vi "欧姆龙PLC初始化FansTCP.vi"() -> (1 "data out":string, 2 "布尔":bool, 3 "TCP网络连接输出":refnum<k5>, 4 "打开TCP连接成功":bool)   [LabVIEW 2014]
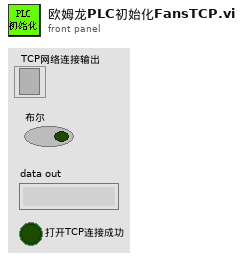
[diagram p1: front panel]
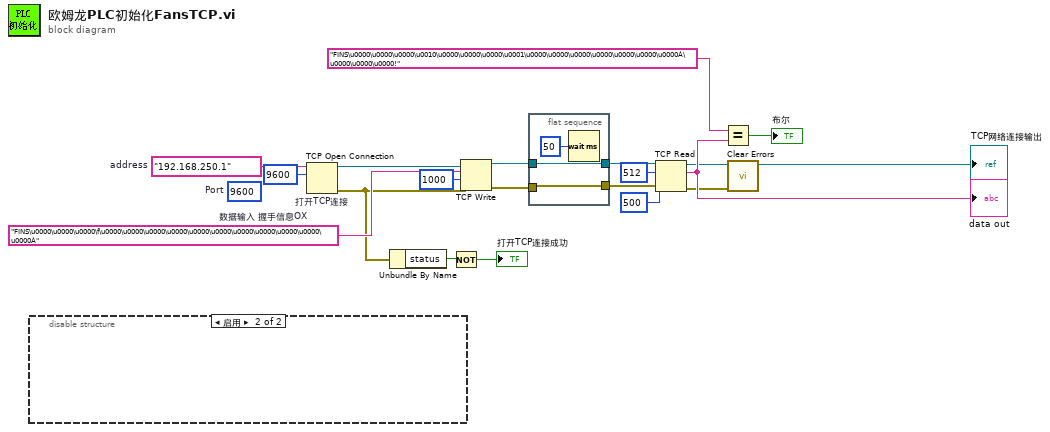
[diagram p0: block diagram]
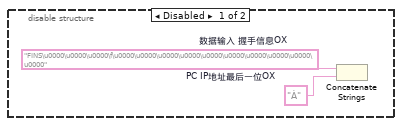
[diagram p2: hidden frame]
diagram:
  w15 = "FINS\u0000\u0000\u0000\f\u0000\u0000\u0000\u0000\u0000\u0000\u0000\u0000\u0000\u0000\u0000À"  # 数据输入 握手信息OX
  (unwired) 9600  # Port
  w2 = "192.168.250.1"  # address
  n1 = disable-structure shown="启用" {
    frame Disabled {
      w21 = "À"  # PC IP地址最后一位OX
      w20 = "FINS\u0000\u0000\u0000\f\u0000\u0000\u0000\u0000\u0000\u0000\u0000\u0000\u0000\u0000"  # 数据输入 握手信息OX
      n2 = Concatenate Strings(w20, w21) -> ()  [unwired: 1 out]
    }
    frame Enabled {
    }
  }
  n3 = TCP Open Connection "打开TCP连接"(address=w2, remote port or service name=u16 9600 ("远程端口或服务名称")) -> (connection ID=w6:refnum<k5>, error out=w7:errorcluster)  [unwired: 3 in]
  n4 = Unbundle By Name(w7) -> ("status"=w5:bool)
  n5 = Not(x=w5) -> (.not. x?=→"打开TCP连接成功":bool)
  n6 = TCP Write(connection ID=w6, data in=w15, error in (no error)=w7, 9:1000 ("超时毫秒(25000)")) -> (connection ID out=w11:refnum<k5>, error out=w9:errorcluster)  [unwired: 1 out]
  n7 = flat-sequence {
    tunnel: w9 -> [w24]
    tunnel: [w24] -> w10
    tunnel: w11 -> [w22]
    tunnel: [w22] -> w12
    frame #0 {
      n8 = Wait (ms)(milliseconds to wait=u32 50 ("等待时间（毫秒）")) -> ()  [unwired: 1 out]
    }
  }
  n9 = TCP Read(connection ID=w12, bytes to read=512 ("读取的字节"), error in (no error)=w10, 9:500 ("超时毫秒(25000)")) -> (connection ID out=→"TCP网络连接输出":refnum<k5>, data out=w19:string, error out=w8:errorcluster)  [unwired: 1 in]
  "data out" <- w19
  n10 = Equal?(x="FINS\u0000\u0000\u0000\u0010\u0000\u0000\u0000\u0001\u0000\u0000\u0000\u0000\u0000\u0000\u0000À\u0000\u0000\u0000!", y=w19) -> (x = y?=→"布尔":bool)
  n11 = call <vilib>:"Clear Errors.vi"("error in (no error)"=w8) -> ()  [unwired: 5 in, 2 out]
